vi "dot_line_dis.vi"(1 "dot pos":cluster{"X":sgl, "Y":sgl}={"X"=100.0, "Y"=100.0}, 2 "line end":cluster{"X":sgl, "Y":sgl}={"X"=100.0, "Y"=100.0}, 3 "line start":cluster{"X":sgl, "Y":sgl}={"X"=100.0, "Y"=100.0}) -> (0 "distance":sgl)   [LabVIEW 2018]
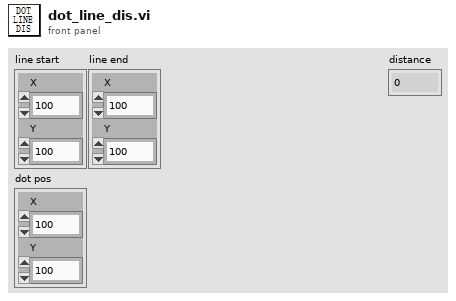
[diagram p1: front panel]
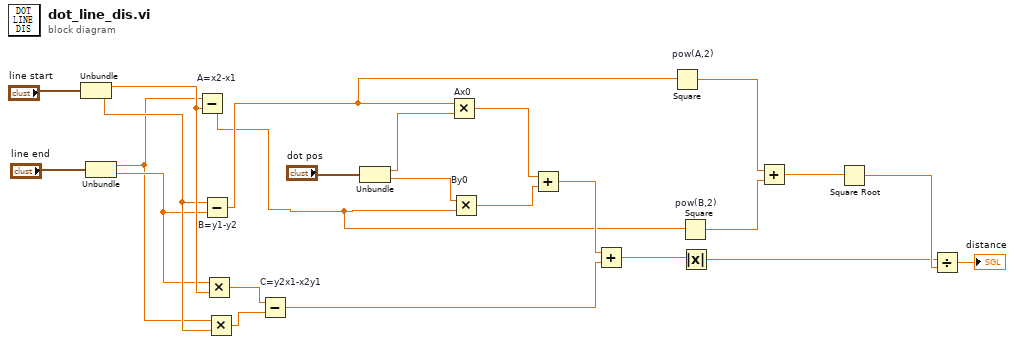
[diagram p0: block diagram]
diagram:
  n1 = Unbundle("line start") -> ("X"=w21:sgl, "Y"=w20:sgl)
  n2 = Unbundle("line end") -> ("X"=w18:sgl, "Y"=w19:sgl)
  n3 = Subtract "A=x2-x1"(x=w18, y=w21) -> (x-y=w1:sgl)
  n4 = Subtract "B=y1-y2"(x=w20, y=w19) -> (x-y=w2:sgl)
  n5 = Multiply(x=w19, y=w21) -> (x*y=w17:sgl)
  n6 = Multiply(x=w18, y=w20) -> (x*y=w16:sgl)
  n7 = Subtract "C=y2x1-x2y1"(x=w17, y=w16) -> (x-y=w10:sgl)
  n8 = Unbundle("dot pos") -> ("X"=w15:sgl, "Y"=w14:sgl)
  n9 = Multiply "Ax0"(x=w2, y=w15) -> (x*y=w13:sgl)
  n10 = Multiply "By0"(x=w14, y=w1) -> (x*y=w12:sgl)
  n11 = Add(x=w13, y=w12) -> (x+y=w11:sgl)
  n12 = Add(x=w11, y=w10) -> (x+y=w4:sgl)
  n13 = Square "pow(A,2)"(x=w2) -> (x^2=w9:sgl)
  n14 = Square "pow(B,2)"(x=w1) -> (x^2=w8:sgl)
  n15 = Absolute Value(x=w4) -> (abs(x)=w3:sgl)
  n16 = Add(x=w9, y=w8) -> (x+y=w7:sgl)
  n17 = Square Root(x=w7) -> (sqrt(x)=w6:sgl)
  n18 = Divide(x=w3, y=w6) -> (x/y=→"distance":sgl)
